vi "Read BLE Message.lvclass.vi"(8 "error in (no error)":errorcluster, 11 "BLE context in":refnum<class "BLE context.lvclass">) -> (0 "error out":errorcluster, 2 "BLE Message.lvclass":refnum<class "BLE Message.lvclass">, 3 "BLE context out":refnum<class "BLE context.lvclass">)   [LabVIEW 2015, in "BLE context.lvclass"]
uses:
  BLE context.lvclass
  BLE Message/BLE Message.lvclass
  BLE context.lvclass/BLE context.ctl
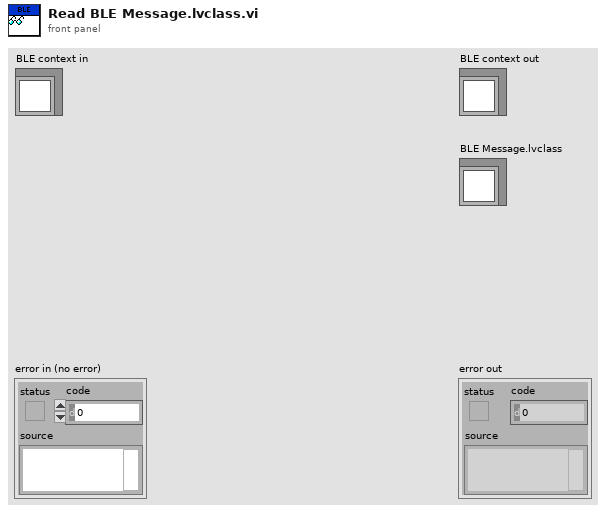
[diagram p1: front panel]
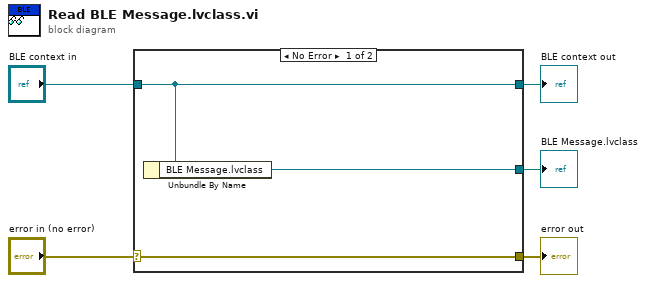
[diagram p0: block diagram]
diagram:
  n1 = case shown="No Error" "error in (no error)" {
    selector: "error in (no error)" -> [w8 w9]
    tunnel: [w8 w9] -> w4
    tunnel: [w7 w10] -> w2
    tunnel: "BLE context in" -> [w7 w10]
    tunnel: [w6 _] -> w1
    frame No Error {
      n2 = Unbundle By Name(w7) -> ("BLE Message.lvclass"=w6:refnum<class "BLE Message.lvclass">)
    }
    frame Error {
    }
  }
  "error out" <- w4
  "BLE context out" <- w2
  "BLE Message.lvclass" <- w1
